vi "PID_Flow Ctrl.vi"(5 "manual":i32, 7 "enable":i32=1, 8 "FrManual":dbl, 9 "Setpoint_T":dbl[](array[numeric])=[2.0, 2.0, 2.0], 10 "Setpoint_W":dbl[](array[numeric])=[10.0, 20.0, 30.0], 11 "weight":dbl) -> (0 "FR":dbl, 1 "step":dbl, 4 "weight":dbl, 6 "RPM":dbl)   [LabVIEW 2016]
uses:
  BERTTA.dll
panel:
  out "count":dbl
  out "Waveform Chart":dbl(graph)
  out "weightChange":dbl
  out "output":dbl
  out "errsum":dbl
  out "error":dbl
  out "setpoint":dbl
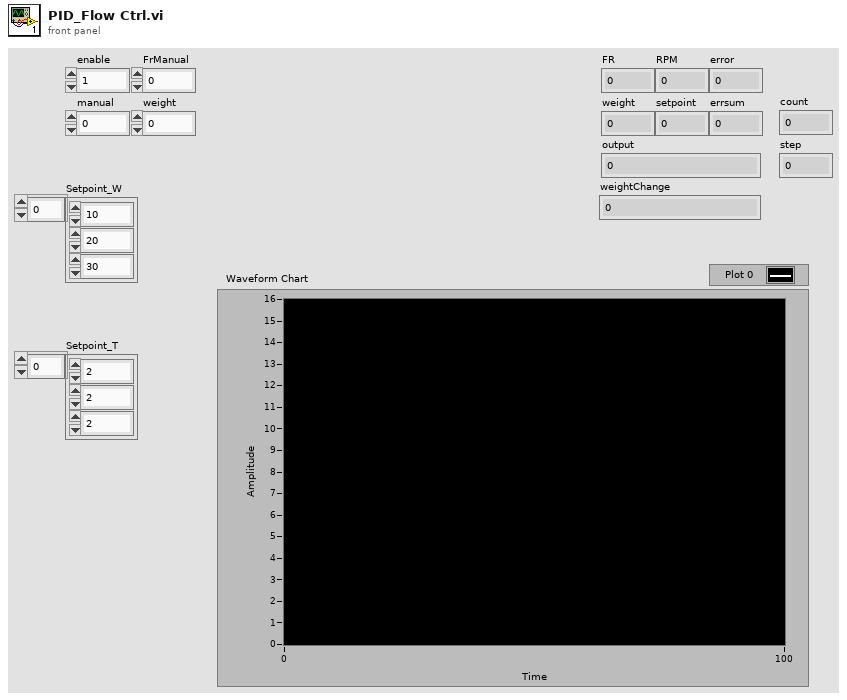
[diagram p1: front panel]
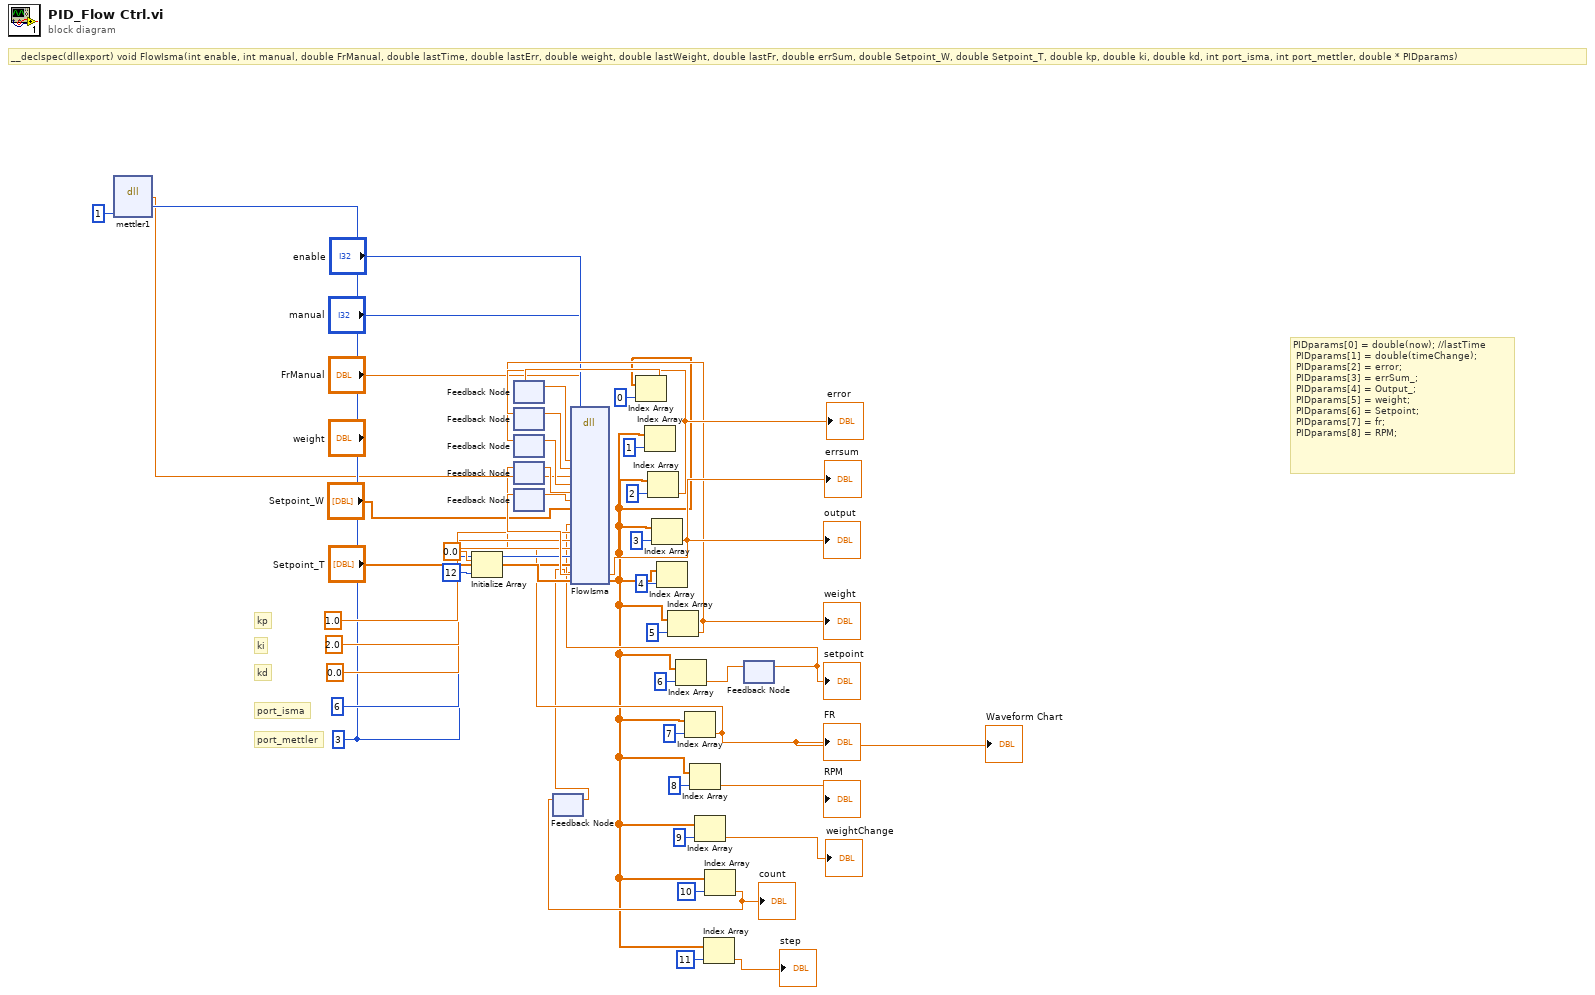
[diagram p0: block diagram]
diagram:
  w15 = 3 ("port_mettler")
  # "port_mettler"
  # "port_isma"
  # "kd"
  # "ki"
  # "kp"
  # "PIDparams[0] = double(now); //lastTime \n\tPIDparams[1] = double(timeChange);\n\tPIDparams[2] = error;\n\tPIDparams[3] = errSum_;\n\tPIDparams[4] = Output_;\n\tPIDparams[5] = weight;\n\tPIDparams[6] = Setpoint;\n\tPIDparams[7] = fr;\n\tPIDparams[8] = RPM;"
  # "__declspec(dllexport) void FlowIsma(int enable, int manual, double FrManual, double lastTime, double lastErr, double weight, double lastWeight, double lastFr, double errSum, double Setpoint_W, double Setpoint_T, double kp, double ki, double kd, int port_isma, int port_mettler, double * PIDparams)"
  n1 = dll-call lib="C:/Users/shresplab/OneDrive - Kemira Oyj/Documents/GitHub/Bertta/BERTTA/x64/Debug/BERTTA.dll" fn="mettler1"("port"=w15, "msg"=1) -> ("return type"=w13:dbl)  [unwired: 5 in, 2 out]
  n2 = Initialize Array(0.0 ("element"), 12 ("dimension size")) -> (w43:dbl[])
  n3 = feedback #1() -> (w32:dbl)  [unwired: 1 in]
  n4 = feedback #2() -> (w30:dbl)  [unwired: 1 in]
  n5 = feedback #3() -> (w26:dbl)  [unwired: 1 in]
  n6 = feedback #4() -> (w25:dbl)  [unwired: 1 in]
  n7 = feedback #5() -> (w28:dbl)  [unwired: 1 in]
  n8 = feedback #6() -> (w4:dbl)  [unwired: 1 in]
  n9 = feedback #7() -> (w7:dbl)  [unwired: 1 in]
  "setpoint" <- w7
  n10 = dll-call lib="C:/Users/shresplab/OneDrive - Kemira Oyj/Documents/GitHub/Bertta/BERTTA/x64/Debug/BERTTA.dll" fn="FlowIsma"("enable"="enable", "manual"="manual", "FrManual"="FrManual", "lastTime"=w32, "lastErr"=w30, "weight"=w13, "lastWeight"=w26, "lastFr"=w25, "errSum"=w28, "Setpoint_W"="Setpoint_W", "Setpoint_T"="Setpoint_T", "lastSP"=w7, "kp"=1.0, "ki"=2.0, "kd"=0.0, "port_isma"=6, "port_mettler"=w15, "count"=w4, "PIDparams"=w43) -> ("PIDparams"=w2:dbl[])  [unwired: 22 in, 2 out]
  n11 = Index Array(array=w2, index=0) -> (element=w33:dbl)
  n12 = feedback-in #1(w33) -> ()
  n13 = Index Array(array=w2, index=1) -> ()  [unwired: 1 out]
  n14 = Index Array(array=w2, index=2) -> (element=w31:dbl)
  "error" <- w31
  n15 = feedback-in #2(w31) -> ()
  n16 = Index Array(array=w2, index=3) -> (element=w29:dbl)
  "errsum" <- w29
  "output" <- w29
  n17 = feedback-in #5(w29) -> ()
  n18 = Index Array(array=w2, index=4) -> ()  [unwired: 1 out]
  n19 = Index Array(array=w2, index=5) -> (element=w27:dbl)
  "weight" <- w27
  n20 = feedback-in #3(w27) -> ()
  n21 = Index Array(array=w2, index=6) -> (element=w8:dbl)
  n22 = Index Array(array=w2, index=7) -> (element=w9:dbl)
  "FR" <- w9
  "Waveform Chart" <- w9
  n23 = feedback-in #4(w9) -> ()
  n24 = Index Array(array=w2, index=8) -> (element=→"RPM":dbl)
  n25 = Index Array(array=w2, index=9) -> (element=→"weightChange":dbl)
  n26 = Index Array(array=w2, index=11) -> (element=→"step":dbl)
  n27 = Index Array(array=w2, index=10) -> (element=w5:dbl)
  "count" <- w5
  n28 = feedback-in #6(w5) -> ()
  n29 = feedback-in #7(w8) -> ()
